vi "RS485ReadNormal.vi"() -> ()   [LabVIEW 2016]
uses:
  <vilib>/Instr/_visa.llb/VISA Configure Serial Port (Instr).vi
panel:
  out "Numeric 2":dbl
  out "Numeric":dbl
  in  "stop":bool
  in  "baud rate":u32=115200
  in  "data bits":u16=8 min=5 max=8 step=1
  in  "parity":u16(ring)=2 items=["None", "Odd", "Even", "Mark", "Space"]
  in  "stop bits":u16(ring)=10 items=["1"=10, "1.5"=15, "2.0"=20]
  in  "flow control":u16(ring) items=["None"=0, "XON/XOFF"=1, "RTS/CTS"=2, "DTR/DSR"=4]
  in  "VISA resource name":refnum<visa-resource-name>="COM4"
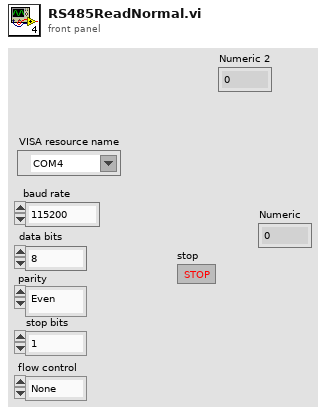
[diagram p1: front panel]
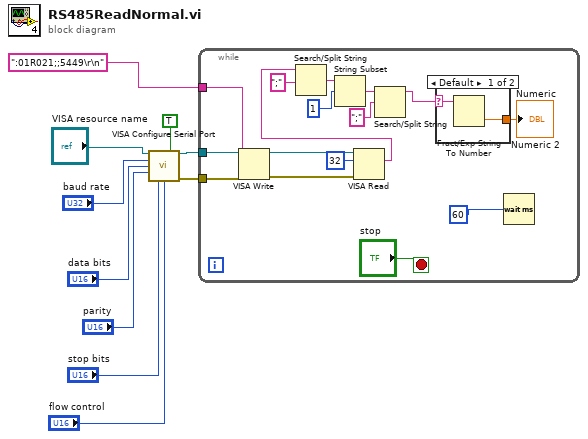
[diagram p0: block diagram]
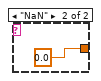
[diagram p2: hidden frame]
diagram:
  n1 = call-poly "VISA Configure Serial Port"("VISA resource name"="VISA resource name", "Enable Termination\nChar (T)"=TRUE, "baud rate (9600)"="baud rate", "data bits (8)"="data bits", "parity (0:none)"="parity", "stop bits (10: 1 bit)"="stop bits", "flow control (0:none)"="flow control") -> ("VISA resource name out"=w8:refnum<visa-resource-name>, "error out"=w9:errorcluster)  [unwired: 7 in]
  n2 = while {
    tunnel: ":01R021;;5449\r\n" ("Command") -> [w25]
    tunnel: w9 -> [w23]
    tunnel: w8 -> [w21]
    stop <- "stop" stop-if-true
    n3 = VISA Write(VISA resource name=w21, write buffer=w25, error in (no error)=w23) -> (VISA resource name out=w22:refnum<visa-resource-name>, error out=w24:errorcluster)  [unwired: 1 out]
    n4 = VISA Read(VISA resource name=w22, byte count=u32 32, error in (no error)=w24) -> (read buffer=w14:string)  [unwired: 3 out]
    n5 = Search/Split String(string=w14, search string/char (-)=";") -> (match + rest of string=w18:string)  [unwired: 1 in, 2 out]
    n6 = String Subset(string=w18, offset (0)=1) -> (substring=w17:string)  [unwired: 1 in]
    n7 = Search/Split String(string=w17, search string/char (-)=";") -> (substring before match=w19:string)  [unwired: 1 in, 2 out]
    n8 = case shown="Default" w19 {
      selector: w19 -> [w28 _]
      tunnel: [w27 0.0] -> w13
      frame Default {
        n9 = Fract/Exp String To Number(string=w28) -> (number=w27:dbl)  [unwired: 3 in, 1 out]
      }
      frame "NaN" {
      }
    }
    "Numeric" <- w13
    n10 = Wait (ms)(milliseconds to wait=60) -> ()  [unwired: 1 out]
  }
